vi "Main_SubVI_Position to Pulse.vi"(8 "Error In":errorcluster, 10 "Postion":dbl, 11 "Axis Number":T1=1 items=["X"=1, "Y"=2, "Z"=3, "Rotation"=4]) -> (0 "Error Out":errorcluster, 3 "Pulse":i32)   [LabVIEW 2015]
uses:
  Control/Control_Axis Number.ctl
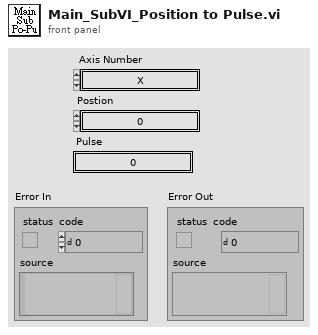
[diagram p1: front panel]
types:
  T1 = typedef "Control_Axis Number.ctl" = u16
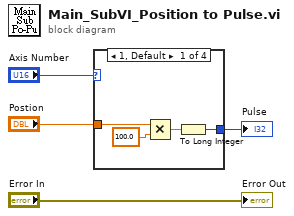
[diagram p0: block diagram]
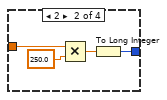
[diagram p2: hidden frame]
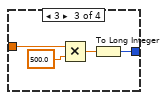
[diagram p3: hidden frame]
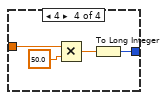
[diagram p4: hidden frame]
diagram:
  n1 = case shown="1, Default" "Axis Number" {
    tunnel: "Postion" -> [w8 w12 w16 w20]
    tunnel: [w5 w9 w13 w17] -> w3
    frame 1, Default {
      n2 = Multiply(x=w8, y=100.0) -> (x*y=w6:dbl)
      n3 = To Long Integer(number=w6) -> (32bit integer=w5:i32)
    }
    frame 2 {
      n4 = Multiply(x=w12, y=250.0) -> (x*y=w10:dbl)
      n5 = To Long Integer(number=w10) -> (32bit integer=w9:i32)
    }
    frame 3 {
      n6 = Multiply(x=w16, y=500.0) -> (x*y=w14:dbl)
      n7 = To Long Integer(number=w14) -> (32bit integer=w13:i32)
    }
    frame 4 {
      n8 = Multiply(x=w20, y=50.0) -> (x*y=w18:dbl)
      n9 = To Long Integer(number=w18) -> (32bit integer=w17:i32)
    }
  }
  "Pulse" <- w3
  "Error Out" <- "Error In"
